vi "Get assoicated LV error for error UIR.vi"(10 "Default error":errorcluster, 11 "URI":string) -> (3 "Associated error":errorcluster)   [LabVIEW 2020, in "wamplv.lvlib"]
uses:
  wamplv.lvlib
  <vilib>/Utility/error.llb/Error Cluster From Error Code.vi
  <vilib>/ErrorRing/Error Ring.xnode
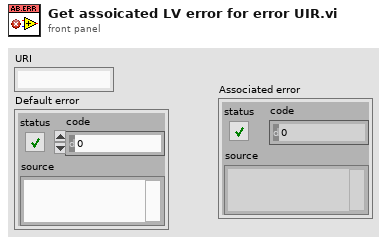
[diagram p1: front panel]
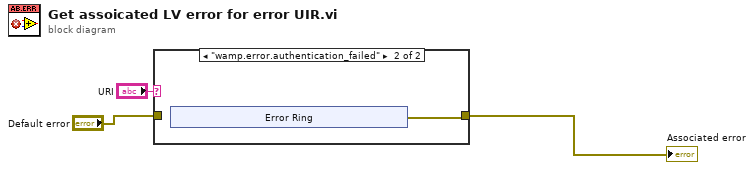
[diagram p0: block diagram]
diagram:
  n1 = case shown="\"wamp.error.authentication_failed\"" "URI" {
    tunnel: [w4 w5] -> w2
    tunnel: "Default error" -> [w4 _]
    frame Default {
    }
    frame "wamp.error.authentication_failed" {
      n2 = xnode "Error Ring"() -> ("error out"=w5:errorcluster)
    }
  }
  "Associated error" <- w2
